vi "Read Error.vi"(8 "error in (no error)":errorcluster, 10 "Key":string, 11 "Item Ref in":T2 format="%.0x") -> (0 "error out":errorcluster, 1 "found?":bool, 2 "VeriStand Error":T1, 3 "Item Ref out":T2 format="%.0x")   [LabVIEW 2015, in "VeriStand Error API.lvlib"]
doc: "<B>Read Error</B> returns the <B>VeriStand Error</B>associated with the given <B>Key</B>"
uses:
  VeriStand Error API.lvlib
  <vilib>/NI Veristand/Custom Device API/Custom Device Item Ref.ctl
  VeriStand Error.ctl
  <vilib>/NI Veristand/Custom Device API/Custom Device API.lvlib
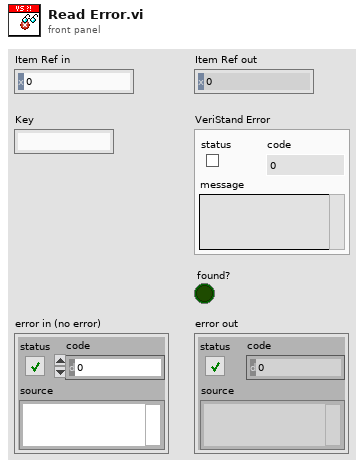
[diagram p1: front panel]
types:
  T1 = typedef "VeriStand Error API.lvlib/VeriStand Error.ctl" = cluster{"status":bool, "code":i32, "message":string}
  T2 = typedef "Custom Device API.lvlib/Custom Device Item Ref.ctl" = u64
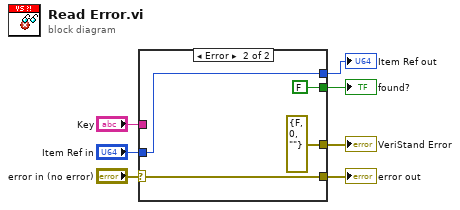
[diagram p0: block diagram]
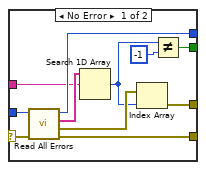
[diagram p2: hidden frame]
diagram:
  n1 = case shown="Error" "error in (no error)" {
    selector: "error in (no error)" -> [w16 w21]
    tunnel: "Item Ref in" -> [w18 w22]
    tunnel: [w17 w22] -> w6
    tunnel: [w15 w21] -> w4
    tunnel: "Key" -> [w13 _]
    tunnel: [w11 T1 {"status"=FALSE, "code"=0, "message"=""} ("VeriStand Error In")] -> w2
    tunnel: [w8 FALSE] -> w1
    frame No Error {
      n2 = call "Read All Errors.vi"("error in (no error)"=w16, "Item Ref in"=w18) -> ("error out"=w15:errorcluster, "VeriStand Errors"=w12:T1[], "Keys"=w14:string[], "Item Ref out"=w17:T2)  [unwired: 6 in]
      n3 = Search 1D Array(1D array=w14, element=w13) -> (index of element=w10:i32)  [unwired: 1 in]
      n4 = Index Array(array=w12, index=w10) -> (element=w11:T1)
      n5 = Not Equal?(x=w10, y=-1) -> (x != y?=w8:bool)
    }
    frame Error {
    }
  }
  "error out" <- w4
  "Item Ref out" <- w6
  "VeriStand Error" <- w2
  "found?" <- w1
